vi "rpc_flash_test.vi"() -> ()   [LabVIEW 2017]
panel:
  in  "string":string
  out "字符串 2":string
  out "error out 2":errorcluster={"status"=TRUE, "code"=56, "source"="UDP Read in UDP.vi->flash.vi"}
  out "Out 2":u8 format="%.0x"
  in  "Firmware":u16(ring)=4 items=["SP6"=4, "Middle"=3, "Final"=2]
  out "Out":u8 format="%.0x"
  in  "Register_Base_Address":u32=512 format="%x"
  in  "Current IP address":string
  in  "error in (no error)":errorcluster
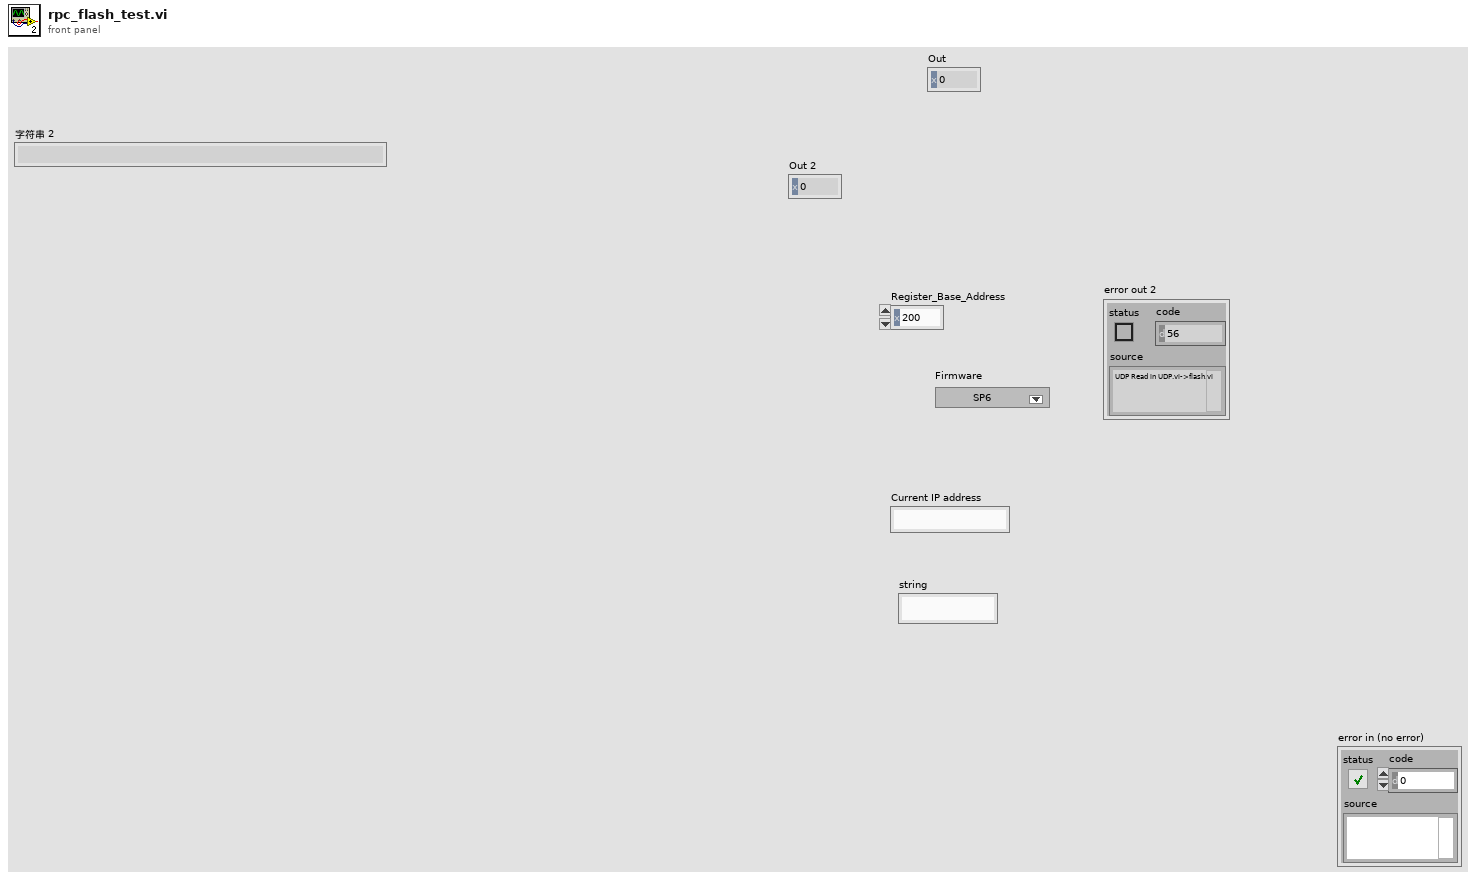
[diagram p1: front panel]
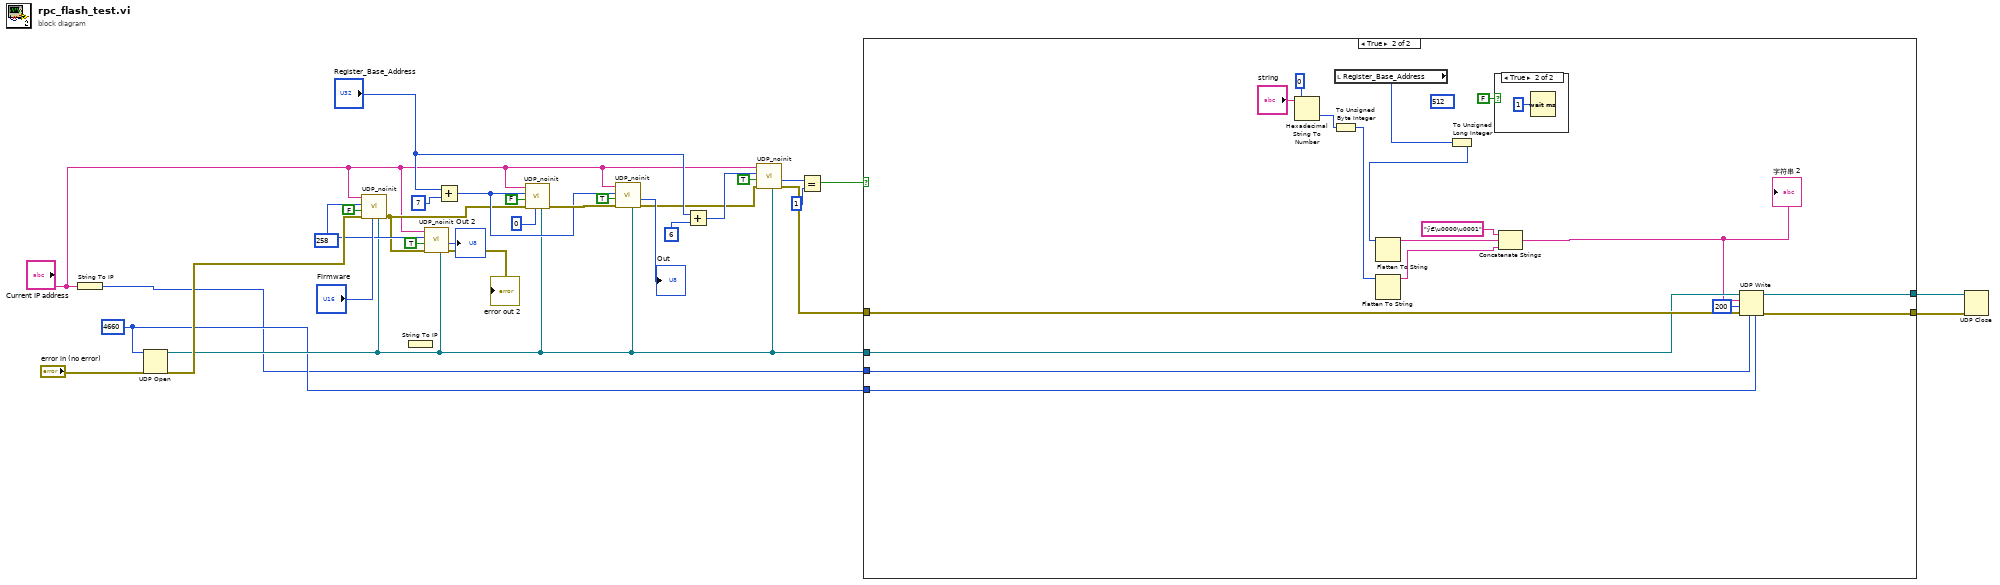
[diagram p0: block diagram]
diagram:
  w18 = u32 258 ("Address")
  w5 = u16 4660 ("UDP port")
  n1 = String To IP(1:"Current IP address") -> (0:w4:u32)
  n2 = UDP Open(8:"error in (no error)", 11:w5) -> (port=w6:refnum<k16>, 0:w19:errorcluster)  [unwired: 3 in, 1 out]
  n3 = call "UDP_noinit.vi"("connection ID"=w6, "In"="Firmware", "error in (no error)"=w19, "Read (TRUE)"=FALSE, "Address"=w18, "IP address"="Current IP address") -> ("error out"=w15:errorcluster)  [unwired: 2 in, 2 out]
  n4 = String To IP() -> ()  [unwired: 1 in, 1 out]
  n5 = call "UDP_noinit.vi"("connection ID"=w6, "error in (no error)"=w15, "Read (TRUE)"=TRUE, "Address"=w18, "IP address"="Current IP address") -> ("error out"=→"error out 2":errorcluster, "Out"=→"Out 2":u8)  [unwired: 3 in, 1 out]
  n6 = Add(x="Register_Base_Address", y=u32 7 ("Address")) -> (x+y=w26:u32)
  n7 = call "UDP_noinit.vi"("connection ID"=w6, "In"=u8 0, "error in (no error)"=w15, "Read (TRUE)"=FALSE, "Address"=w26, "IP address"="Current IP address") -> ("error out"=w29:errorcluster)  [unwired: 2 in, 2 out]
  n8 = call "UDP_noinit.vi"("connection ID"=w6, "error in (no error)"=w29, "Read (TRUE)"=TRUE, "Address"=w26, "IP address"="Current IP address") -> ("error out"=w2:errorcluster, "Out"=→"Out":u8)  [unwired: 3 in, 1 out]
  n9 = Add(x="Register_Base_Address", y=u32 6 ("Address")) -> (x+y=w10:u32)
  n10 = call "UDP_noinit.vi"("connection ID"=w6, "error in (no error)"=w2, "Read (TRUE)"=TRUE, "Address"=w10, "IP address"="Current IP address") -> ("error out"=w1:errorcluster, "Out"=w12:u8)  [unwired: 3 in, 1 out]
  n11 = Equal?(x=w12, y=u8 1) -> (x = y?=w9:bool)
  n12 = case shown="True" w9 {
    tunnel: w1 -> [w32 w42]
    tunnel: [w32 w41] -> w8
    tunnel: [w33 w40] -> w7
    tunnel: w6 -> [w33 w39]
    tunnel: w5 -> [_ w36]
    tunnel: w4 -> [_ w35]
    frame False {
    }
    frame True {
      (unwired) u32 512 ("Address")
      n13 = Hexadecimal String To Number(string="string", default (0uL)=u64 0 ("default (0 U32)")) -> (number=w49:u64)  [unwired: 1 in, 1 out]
      n14 = To Unsigned Byte Integer(number=w49) -> (unsigned 8bit integer=w48:u8)
      n15 = local read "Register_Base_Address"() -> (w43:u32)
      n16 = Flatten To String(anything=w48) -> (data string=w44:string)  [unwired: 3 in, 2 out]
      n17 = To Unsigned Long Integer(number=w43) -> (unsigned 32bit integer=w47:u32)
      n18 = Flatten To String(anything=w47) -> (data string=w45:string)  [unwired: 3 in, 2 out]
      n19 = case shown="True" FALSE {
        frame False {
        }
        frame True {
          n20 = Wait (ms)(milliseconds to wait=u32 1) -> ()  [unwired: 1 out]
        }
      }
      n21 = Concatenate Strings("ÿ€\u0000\u0001" ("initial string"), w45, w44) -> (w38:string)
      "字符串 2" <- w38
      n22 = UDP Write(address=w35, port or service name=w36, connection ID=w39, data in=w38, 8:w42, 9:200 ("timeout ms (25000)")) -> (error out=w41:errorcluster, 3:w40:refnum<k16>)
    }
  }
  n23 = UDP Close(connection ID=w7, 8:w8) -> ()  [unwired: 2 out]
